vi "group_1_donottouch.vi"() -> ()   [LabVIEW 2014]
uses:
  <vilib>/Utility/file.llb/Write To Spreadsheet File (DBL).vi
panel:
  out "Numeric 2":dbl
  out "Numeric":dbl
  out "XY Graph":cluster{dbl[], dbl[]}(graph)
  in  "stop":bool
  in  "I":dbl
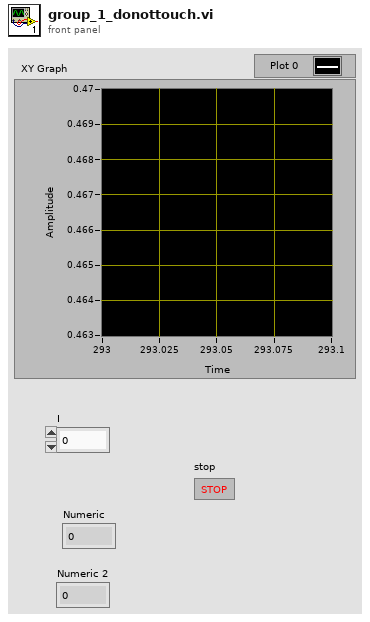
[diagram p1: front panel]
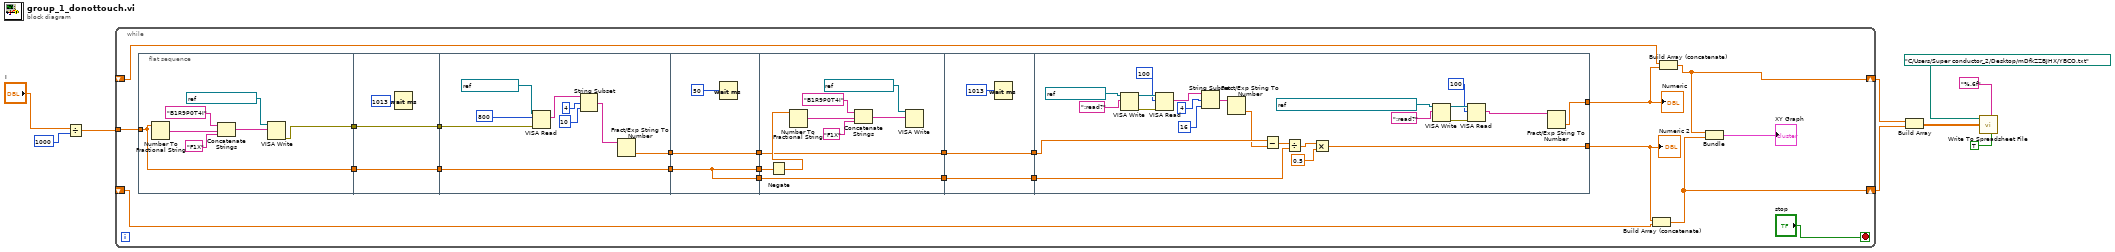
[diagram p0: block diagram]
diagram:
  n1 = Divide(x="I", y=1000) -> (x/y=w7:dbl)
  n2 = while {
    tunnel: w7 -> [w31]
    shift-right: [w17] -> w5
    shift-left: _ -> [w14]
    shift-right: [w16] -> w6
    shift-left: _ -> [w15]
    stop <- "stop" stop-if-true
    n3 = flat-sequence {
      tunnel: w31 -> [w32]
      tunnel: [w33] -> w29
      tunnel: [w32] -> w28
      tunnel: [w40] -> w30
      tunnel: w29 -> [w40]
      tunnel: w28 -> [w39]
      tunnel: [w39] -> w27
      tunnel: w30 -> [w49]
      tunnel: w27 -> [w43]
      tunnel: [w43] -> w26
      tunnel: [w42] -> w21
      tunnel: w26 -> [w51]
      tunnel: [w51] -> w25
      tunnel: [w52] -> w22
      tunnel: w21 -> [w52]
      tunnel: [w51] -> w19
      tunnel: w25 -> [w56]
      tunnel: [w55] -> w23
      tunnel: w22 -> [w55]
      tunnel: [w54] -> w20
      tunnel: w19 -> [w54]
      tunnel: [w64] -> w24
      tunnel: w23 -> [w64]
      tunnel: w20 -> [w63]
      tunnel: [w63] -> w18
      tunnel: w24 -> [w67]
      tunnel: w18 -> [w78]
      tunnel: [w69] -> w11
      tunnel: [w68] -> w10
      frame #0 {
        n4 = Number To Fractional String(number=w32) -> (F-format string=w38:string)  [unwired: 3 in]
        n5 = Concatenate Strings("B1R9P0T4I", w38, "F1X") -> (w35:string)
        n6 = VISA Write(VISA resource name=refnum<visa-resource-name> "GPIB0::12::INSTR", write buffer=w35) -> (error out=w33:errorcluster)  [unwired: 1 in, 2 out]
      }
      frame #1 {
        n7 = Wait (ms)(milliseconds to wait=1013) -> ()  [unwired: 1 out]
      }
      frame #2 {
        n8 = VISA Read(VISA resource name=refnum<visa-resource-name> "GPIB0::15::INSTR", byte count=800, error in (no error)=w49) -> (read buffer=w48:string)  [unwired: 3 out]
        n9 = String Subset(string=w48, offset (0)=4, length (rest)=10) -> (substring=w45:string)
        n10 = Fract/Exp String To Number(string=w45) -> (number=w42:dbl)  [unwired: 3 in, 1 out]
      }
      frame #3 {
        n11 = Wait (ms)(milliseconds to wait=50) -> ()  [unwired: 1 out]
      }
      frame #4 {
        n12 = Negate(x=w56) -> (-x=w57:dbl)
        n13 = Number To Fractional String(number=w57) -> (F-format string=w62:string)  [unwired: 3 in]
        n14 = Concatenate Strings("B1R9P0T4I", w62, "F1X") -> (w59:string)
        n15 = VISA Write(VISA resource name=refnum<visa-resource-name> "GPIB0::12::INSTR", write buffer=w59) -> ()  [unwired: 1 in, 3 out]
      }
      frame #5 {
        n16 = Wait (ms)(milliseconds to wait=1013) -> ()  [unwired: 1 out]
      }
      frame #6 {
        n17 = VISA Write(VISA resource name=refnum<visa-resource-name> "GPIB0::15::INSTR", write buffer=":read?") -> (VISA resource name out=w85:refnum<visa-resource-name>, error out=w86:errorcluster)  [unwired: 1 in, 1 out]
        n18 = VISA Read(VISA resource name=w85, byte count=100, error in (no error)=w86) -> (read buffer=w83:string)  [unwired: 3 out]
        n19 = String Subset(string=w83, offset (0)=4, length (rest)=16) -> (substring=w80:string)
        n20 = Fract/Exp String To Number(string=w80) -> (number=w66:dbl)  [unwired: 3 in, 1 out]
        n21 = Subtract(x=w67, y=w66) -> (x-y=w79:dbl)
        n22 = Divide(x=w79, y=w78) -> (x/y=w77:dbl)
        n23 = Multiply(x=w77, y=0.5) -> (x*y=w68:dbl)
        n24 = VISA Write(VISA resource name=refnum<visa-resource-name> "GPIB0::27::INSTR", write buffer=":read?") -> (VISA resource name out=w72:refnum<visa-resource-name>, error out=w73:errorcluster)  [unwired: 1 in, 1 out]
        n25 = VISA Read(VISA resource name=w72, byte count=100, error in (no error)=w73) -> (read buffer=w70:string)  [unwired: 3 out]
        n26 = Fract/Exp String To Number(string=w70) -> (number=w69:dbl)  [unwired: 3 in, 1 out]
      }
    }
    n27 = Build Array (concatenate)(w10, w14) -> (w17:dbl[])
    n28 = Build Array (concatenate)(w15, w11) -> (w16:dbl[])
    n29 = Bundle(w16, w17) -> (→"XY Graph":cluster{dbl[], dbl[]})  [unwired: 1 in]
    "Numeric" <- w11
    "Numeric 2" <- w10
  }
  n30 = Build Array(w6, w5) -> (w3:dbl[][])
  n31 = call-poly <vilib>:"Write To Spreadsheet File.vi"("transpose? (no:F)"=TRUE, "format (%.3f)"="%.6f", "2D data"=w3, "file path (dialog if empty)"=path "C:/Users/Super conductor_2/Desktop/mDfkZZBJHX/YBCO.txt") -> ()  [unwired: 4 in, 1 out]
